vi "Configure TCPIP Session.vi"(7 "config file name":string, 8 "error in (no error)":errorcluster, 11 "TCPIP Communications in":refnum<class "TCPIP Communications.lvclass">) -> (0 "error out":errorcluster, 3 "TCPIP Communications out":refnum<class "TCPIP Communications.lvclass">)   [LabVIEW 2015, in "TCPIP Communications Framework.lvlib" / "TCPIP Communications.lvclass"]
uses:
  TCPIP Communications.lvclass
  TCPIP Communications.lvclass/TCPIP Communications.ctl
  <vilib>/Utility/config.llb/Read Key (String).vi
  <vilib>/Utility/config.llb/Read Key (U32).vi
  <vilib>/Utility/config.llb/Read Key (I32).vi
  <vilib>/Utility/config.llb/NI_LVConfig.lvlib
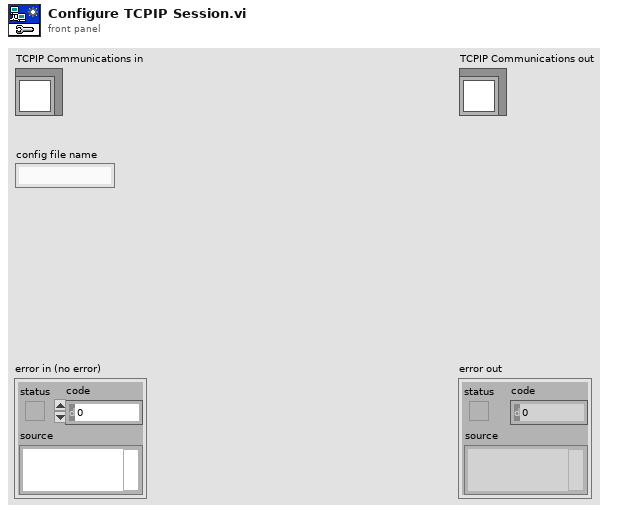
[diagram p1: front panel]
types:
  T1 = typedef "NI_LVConfig.lvlib/Config Data RefNum.ctl" = refnum<k1>
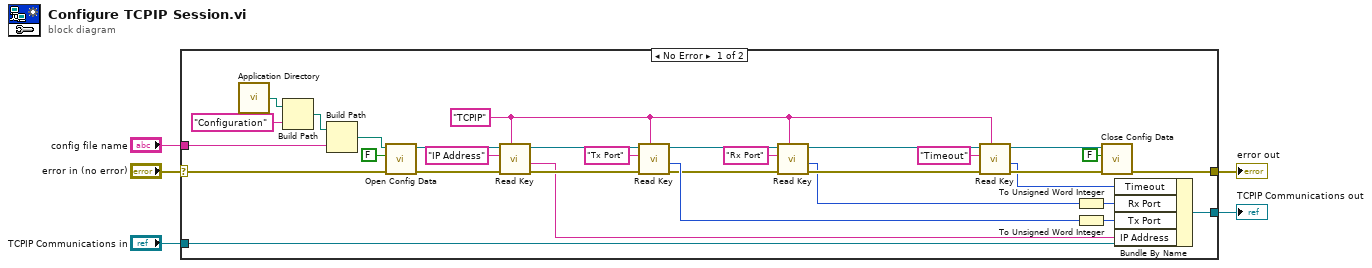
[diagram p0: block diagram]
diagram:
  n1 = case shown="No Error" "error in (no error)" {
    selector: "error in (no error)" -> [w29 w39]
    tunnel: [w21 w39] -> w4
    tunnel: [w24 w38] -> w2
    tunnel: "TCPIP Communications in" -> [w37 w38]
    tunnel: "config file name" -> [w6 _]
    frame No Error {
      w10 = "TCPIP" ("section")
      n2 = call <vilib>:"Application Directory.vi"() -> ("Application Directory"=w32:path)
      n3 = Build Path(base path=w32, name or relative path="Configuration") -> (appended path=w30:path)
      n4 = Build Path(base path=w30, name or relative path=w6) -> (appended path=w34:path)
      n5 = call <vilib>:"Open Config Data.vi"("error in (no error)"=w29, "create file if necessary (T)"=FALSE, "configuration file path"=w34) -> ("error out"=w36:errorcluster, "refnum"=w35:T1)  [unwired: 6 in, 1 out]
      n6 = call-poly <vilib>:"Read Key.vi"("section"=w10, "error in (no error)"=w36, "key"="IP Address", "refnum"=w35) -> ("error out"=w26:errorcluster, "value"=w22:string, "refnum out"=w27:T1)  [unwired: 4 in, 1 out]
      n7 = call-poly <vilib>:"Read Key.vi"("section"=w10, "error in (no error)"=w26, "key"="Tx Port", "refnum"=w27) -> ("error out"=w13:errorcluster, "value"=w23:u32, "refnum out"=w12:T1)  [unwired: 4 in, 1 out]
      n8 = call-poly <vilib>:"Read Key.vi"("section"=w10, "error in (no error)"=w13, "key"="Rx Port", "refnum"=w12) -> ("error out"=w14:errorcluster, "value"=w7:u32, "refnum out"=w11:T1)  [unwired: 4 in, 1 out]
      n9 = call-poly <vilib>:"Read Key.vi"("section"=w10, "error in (no error)"=w14, "key"="Timeout", "refnum"=w11) -> ("error out"=w19:errorcluster, "value"=w16:i32, "refnum out"=w18:T1)  [unwired: 4 in, 1 out]
      n10 = To Unsigned Word Integer(number=w7) -> (unsigned 16bit integer=w8:u16)
      n11 = To Unsigned Word Integer(number=w23) -> (unsigned 16bit integer=w9:u16)
      n12 = call <vilib>:"Close Config Data.vi"("error in (no error)"=w19, "write file if changed (T)"=FALSE, "refnum"=w18) -> ("error out"=w21:errorcluster)  [unwired: 7 in, 1 out]
      n13 = Bundle By Name(cluster=w37, "Timeout"=w16, "Rx Port"=w8, "Tx Port"=w9, "IP Address"=w22) -> (w24:refnum<class "TCPIP Communications.lvclass">)
    }
    frame Error {
    }
  }
  "error out" <- w4
  "TCPIP Communications out" <- w2
